vi "Client (simple).vi"() -> ()   [LabVIEW 2020]
uses:
  Globals and TypeDefs/StationVIReference.ctl
panel:
  out "?":cluster{dbl[]}[](graph)
  in  "Action Control":i32
  out "messages":string
  in  "host:station":string
  out "StationVIReference":T1
  out "error out":errorcluster
  in  "error in (no error)":errorcluster
  out "plot name":string
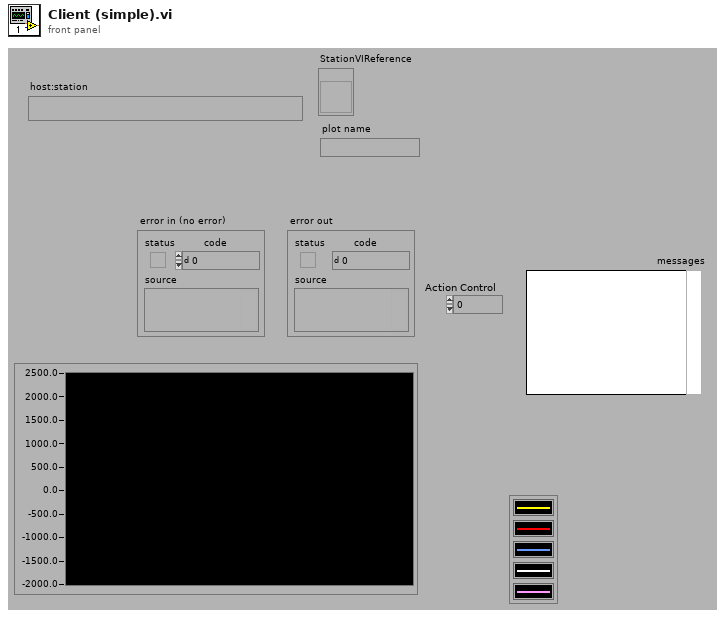
[diagram p1: front panel]
types:
  T1 = typedef "StationVIReference.ctl" = refnum<vi>
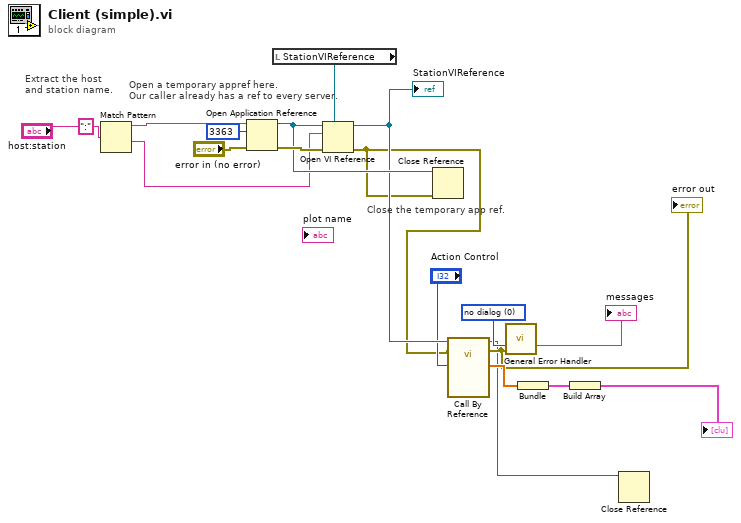
[diagram p0: block diagram]
diagram:
  w13 = u16 0 items=["no dialog", "OK message", "continue or stop message"] ("type of dialog (OK msg:1)")
  # "Open a temporary appref here.\nOur caller already has a ref to every server."
  # "Close the temporary app ref."
  # "Extract the host\nand station name."
  n1 = Match Pattern(string="host:station", regular expression=":") -> (before substring=w3:string, after substring=w2:string)  [unwired: 1 in, 2 out]
  n2 = Open Application Reference(8:"error in (no error)", 10:u32 3363 ("port number (3363)"), 11:w3) -> (0:w15:errorcluster, 3:w14:refnum<vi>)  [unwired: 1 in]
  n3 = local read "StationVIReference"() -> (w16:T1)
  n4 = Open VI Reference(type specifier VI Refnum (for type only)=w16, application reference (local)=w14, vi path=w2, error in (no error)=w15) -> (vi reference=w11:T1, error out=w9:errorcluster)  [unwired: 2 in]
  "StationVIReference" <- w11
  n5 = Close Reference(reference=w14, error in (no error)=w9) -> ()  [unwired: 1 out]
  n6 = call-by-ref "?"(reference=w11, error in=w9, "phase"="Action Control") -> (reference out=w4:T1, error out=w5:errorcluster, 3:w12:dbl[])  [unwired: 6 in]
  "error out" <- w5
  n7 = call <vilib>:"General Error Handler.vi"("type of dialog (OK msg:1)"=w13, "error in (no error)"=w5) -> ("message"=→"messages":string)  [unwired: 9 in, 4 out]
  n8 = Bundle(w12) -> (w7:cluster{dbl[]})  [unwired: 1 in]
  n9 = Build Array(w7) -> (→"?":cluster{dbl[]}[])
  n10 = Close Reference(reference=w4) -> ()  [unwired: 1 in, 1 out]
